vi "add_int64_roslv.vi"   [LabVIEW 2014]
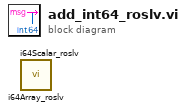
[diagram p0: block diagram]
diagram:
  n1 = call "i64Array_roslv.vi"() -> ()  [unwired: 5 in, 1 out]
  n2 = call "i64Scalar_roslv.vi"() -> ()  [unwired: 5 in, 1 out]
